vi "Check CMD Starts.vi"(7 "Controller Type:":T1, 9 "Last CMDs":dbl[](array[numeric]), 10 "Current CMDs":dbl[](array[numeric]), 11 "Restarts Cluster IN":T2={"CMD Starts:"=[0, 0, 0, 0, 0, 0], "Restarts:"=[0, 0, 0, 0, 0, 0], "Total CMD:"=[0, 0, 0, 0, 0, 0], "Total Restarts:"=[0, 0, 0, 0, 0, 0]}) -> (3 "Restarts Cluster OUT":T2)   [LabVIEW 2019]
uses:
  Type Defs/Restarts Cluster.ctl
  Type Defs/Controller Names.ctl
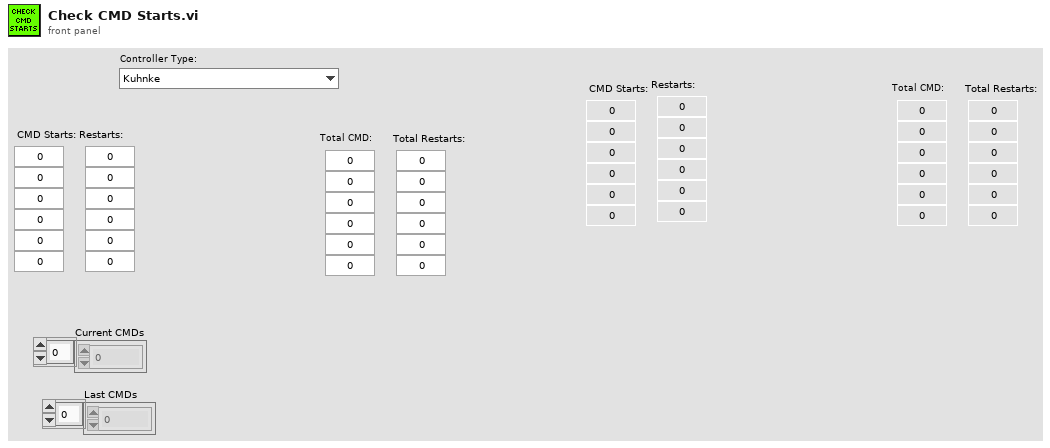
[diagram p1: front panel]
types:
  T1 = typedef "Controller Names.ctl" = enum16{"Kuhnke", "Conti", "Hella BLDC OL PWM", "Hella BLDC Turbine OL PWM", "Helbako", "TI PWM", "PSA", "Hella DC Gas", "Hella DC Diesel", "8 Comm", "10 Comm", "8 Comm Hella", "10 Comm Hella", "8 Comm Omron", "10 Comm Omron", "8 Comm Nissan", "10 Comm Nissan", "TI HP BLDC", "Mazda BLDC"}
  T2 = typedef "Restarts Cluster.ctl" = cluster{"CMD Starts:":i32[], "Restarts:":i32[], "Total CMD:":i32[], "Total Restarts:":i32[]}
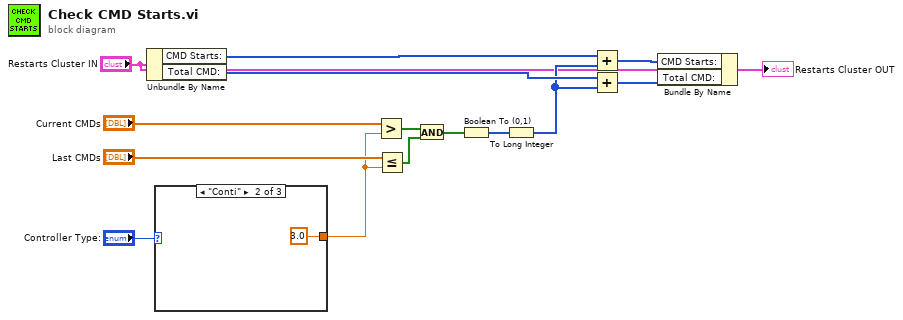
[diagram p0: block diagram]
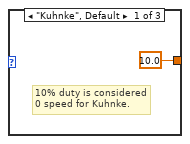
[diagram p2: hidden frame]
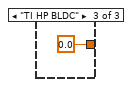
[diagram p3: hidden frame]
diagram:
  n1 = Unbundle By Name("Restarts Cluster IN") -> ("CMD Starts:"=w8:i32[], "Total CMD:"=w7:i32[])
  n2 = case shown="\"Conti\"" "Controller Type:" {
    tunnel: [10.0 3.0 0.0] -> w11
    frame "Kuhnke", Default {
      # "10% duty is considered\n0 speed for Kuhnke."
    }
    frame "Conti" {
    }
    frame "TI HP BLDC" {
    }
  }
  n3 = Greater?(x="Current CMDs", y=w11) -> (0:w10:bool[])
  n4 = Less Or Equal?(x="Last CMDs", y=w11) -> (x <= y?=w9:bool[])
  n5 = And(x=w10, y=w9) -> (x .and. y?=w15:bool[])
  n6 = Boolean To (0,1)(Boolean=w15) -> (0, 1=w14:i16[])
  n7 = To Long Integer(number=w14) -> (32bit integer=w6:i32[])
  n8 = Add(x=w8, y=w6) -> (x+y=w4:i32[])
  n9 = Add(x=w7, y=w6) -> (x+y=w3:i32[])
  n10 = Bundle By Name(cluster="Restarts Cluster IN", "CMD Starts:"=w4, "Total CMD:"=w3) -> (→"Restarts Cluster OUT":T2)
